vi "svc_Complex Array to Polar or Rectangular Components.vi"(2 "View":enum16{"Mag-Phase", "Real-Imaginary"}(ring), 4 "complex array":cdb[](array[numeric]) format="%.2f") -> (0 "phase or imaginary part":dbl[](array[numeric]) format="%.2f", 1 "magnitude or real part":dbl[](array[numeric]) format="%.2f")   [LabVIEW 2017]
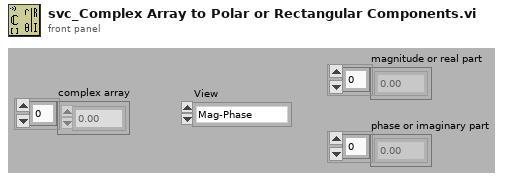
[diagram p1: front panel]
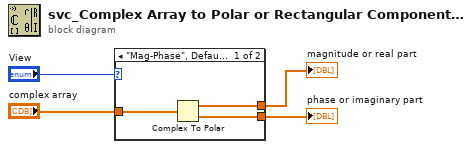
[diagram p0: block diagram]
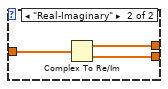
[diagram p2: hidden frame]
diagram:
  n1 = case shown="\"Mag-Phase\", Default" "View" {
    tunnel: "complex array" -> [w7 w10]
    tunnel: [w6 w9] -> w4
    tunnel: [w5 w8] -> w3
    frame "Mag-Phase", Default {
      n2 = Complex To Polar(r * e^(i*theta)=w7) -> (r=w6:dbl[], theta=w5:dbl[])
    }
    frame "Real-Imaginary" {
      n3 = Complex To Re/Im(x + iy=w10) -> (x=w9:dbl[], y=w8:dbl[])
    }
  }
  "magnitude or real part" <- w4
  "phase or imaginary part" <- w3
